vi "SystemGetState.vi"(8 "error in (no error)":errorcluster {"code" format="%.0x"}, 9 "pDataBufferSize":i32=2048 caption="pDataBufferSize (2048)", 11 "instrument handle":refnum<k15>) -> (0 "error out":errorcluster {"code" format="%.0x"}, 1 "pDataActualSize":i32, 2 "pData":string, 3 "instrument handle out":refnum<k15>)   [LabVIEW 2009, in "Keysight XSAn.lvlib"]
doc: "Binary current instrument state. May be restored using PutState method. Data is in internal instrument format, do not alter.\n\nSupported Models: All supported"
uses:
  <instrlib>/Keysight XSAn/Keysight XSAn.lvlib
  AgXSAn.dll
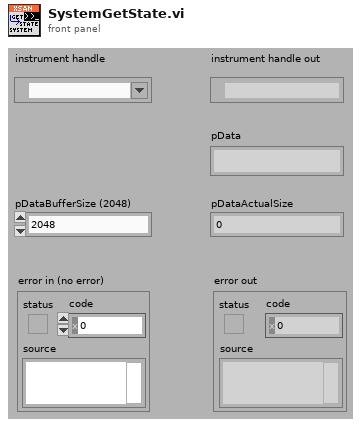
[diagram p1: front panel]
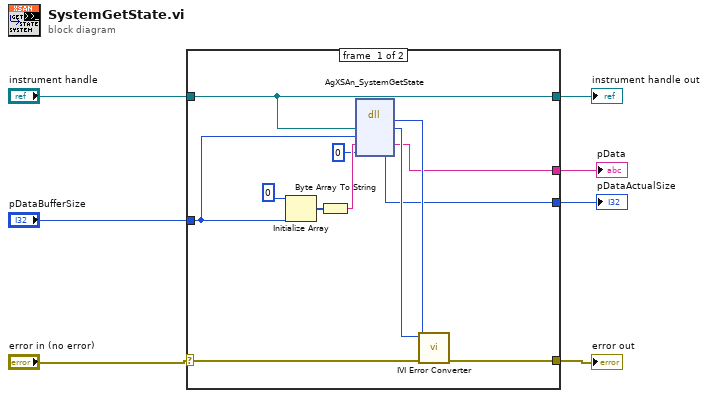
[diagram p0: block diagram]
diagram:
  n1 = case shown="No Error" "error in (no error)" {
    selector: "error in (no error)" -> [w17 w21]
    tunnel: [w16 w21] -> w7
    tunnel: "instrument handle" -> [w9 w20]
    tunnel: "pDataBufferSize" -> [w8 _]
    tunnel: [w12 _] -> w3
    tunnel: [w10 _] -> w2
    tunnel: [w9 w20] -> w1
    frame #0 {
      n2 = Initialize Array(u8 0 ("element"), w8) -> (w14:u8[])
      n3 = Byte Array To String(unsigned byte array=w14) -> (string=w15:string)
      n4 = dll-call lib="AgXSAn**.dll" fn="AgXSAn_SystemGetState"("Vi"=w9, "pDataBufferSize"=w8, "pData"=w15, "pDataActualSize"=0) -> (w18:i32, "Vi"=w19:u32, "pData"=w12:string, "pDataActualSize"=w10:i32)  [unwired: 4 in, 2 out]
      n5 = call <instrlib>:"IVI Error Converter.vi"("error in (no error)"=w17, "IVI error code (0)"=w18, "instrument handle"=w19) -> ("error out"=w16:errorcluster)  [unwired: 7 in, 1 out]
    }
    frame #1 {
    }
  }
  "error out" <- w7
  "instrument handle out" <- w1
  "pData" <- w3
  "pDataActualSize" <- w2
